vi "testLuaYield.vi"() -> ()   [LabVIEW 2011]
uses:
  wrapper/lua_yieldP/lua_repacked.dll
panel:
  out "lua_State *luaL_newstate":u64
  out "lua_yieldk":i32(ring) items=["LUA_OK", "LUA_YIELD", "LUA_ERRRUN", "LUA_ERRSYNTAX", "LUA_ERRMEM", "LUA_ERRGCMM", "LUA_ERRERR"]
  out "数值":i32
  in  "停止":bool
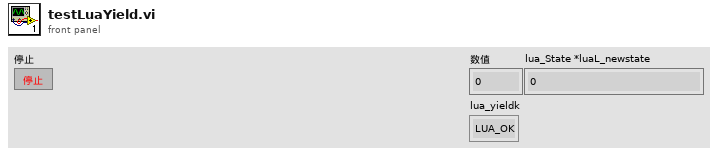
[diagram p1: front panel]
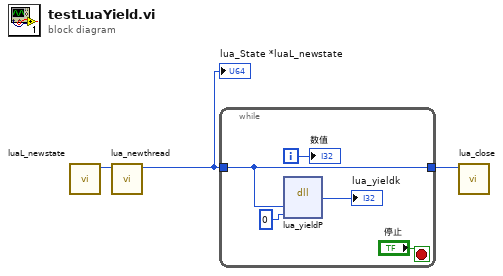
[diagram p0: block diagram]
diagram:
  n1 = call "luaL_newstate.vi"() -> ("lua_State *luaL_newstate"=w2:u64)  [unwired: 10 in, 1 out]
  n2 = call "lua_newthread.vi"("lua_State *L"=w2) -> ("lua_State *lua_newthread"=w1:u64)  [unwired: 9 in, 1 out]
  "lua_State *luaL_newstate" <- w1
  n3 = while {
    tunnel: w1 -> [w5]
    tunnel: [w5] -> w3
    i -> [w7]
    stop <- "停止" stop-if-true
    n4 = dll-call lib="G:/work/Training System 2011/monkey task 2012/source program/LuaDllToLabview/wrapper/lua_yieldP/lua_repacked.dll" fn="lua_yieldP"("lua_State *L"=w5, "n"=0 ("nresults")) -> ("lua_yieldP"=→"lua_yieldk":i32)  [unwired: 5 in, 2 out]
    "数值" <- w7
  }
  n5 = call "lua_close.vi"("lua_State *L"=w3) -> ()  [unwired: 10 in, 1 out]
